vi "IRcam check.vi"() -> ()   [LabVIEW 2021]
uses:
  <vilib>/Platform/TimedLoop/XDataNode/timing_clust.ctl
  <vilib>/Platform/TimedLoop/XDataNode/nitl_modes.ctl
  <vilib>/Platform/TimedLoop/XDataNode/wakeup.ctl
  <vilib>/myRIO/Instrument Drivers/Onboard IO/I2C/typedefs/I2C User Configuration.ctl
  <vilib>/myRIO/Instrument Drivers/Onboard IO/I2C/typedefs/I2C Transfer Rate.ctl
  <vilib>/myRIO/Instrument Drivers/Onboard IO/I2C/typedefs/I2C Reference.ctl
  <vilib>/myRIO/Common/Instrument Driver Framework/Utilities/typedefs/myRIO Generic Hardware Reference.ctl
  <vilib>/myRIO/Common/Instrument Driver Framework/Utilities/typedefs/Hardware Version Enum.ctl
  <vilib>/myRIO/Common/Instrument Driver Framework/Utilities/typedefs/myRIO v1.0 Reference.ctl
  <vilib>/myRIO/Common/Instrument Driver Framework/Utilities/typedefs/Generic FPGA Reference.ctl
  <vilib>/myRIO/Common/Instrument Driver Framework/myRIO v1.0/I2C/typedefs/I2C Channels Enum.ctl
  <vilib>/myRIO/Instrument Drivers/Onboard IO/I2C/typedefs/I2C Configuration.ctl
  <vilib>/userDefined/High Color/nirio_resource_hc.ctl
  <vilib>/myRIO/Common/Instrument Driver Framework/Utilities/vis/Is FPGA Ref Available.vi
  <vilib>/myRIO/Common/Instrument Driver Framework/myRIO v1.0/I2C/vis/myRIO v1.1 Open I2C.vi
  <vilib>/myRIO/Instrument Drivers/Onboard IO/I2C/vis/Configure.vi
  <vilib>/myRIO/Instrument Drivers/Onboard IO/I2C/vis/Write.vi
  <vilib>/myRIO/Instrument Drivers/Onboard IO/I2C/vis/Write Read.vi
  <vilib>/myRIO/Common/Instrument Driver Framework/Utilities/vis/Validate Channels.vi
  <vilib>/myRIO/Common/Instrument Driver Framework/myRIO v1.0/I2C/vis/myRIO v1.0 Reserve I2C.vi
  <vilib>/myRIO/Common/Instrument Driver Framework/myRIO v1.0/I2C/vis/myRIO v1.0 Build MUX Configuration I2C.vi
  <vilib>/myRIO/Common/Instrument Driver Framework/myRIO v1.0/Resource Manager/vis/myRIO v1.0 Reserve Channel List.vi
  <vilib>/myRIO/Common/Instrument Driver Framework/myRIO v1.0/Resource Manager/vis/myRIO v1.0 Create Configuration List.vi
  <vilib>/myRIO/Common/Instrument Driver Framework/myRIO v1.0/Resource Manager/vis/myRIO v1.0 Reserve Channel.vi
  <vilib>/myRIO/Common/Instrument Driver Framework/myRIO v1.0/Resource Manager/vis/myRIO v1.0 Unreserve Channel.vi
  <vilib>/myRIO/Common/Instrument Driver Framework/myRIO v1.0/Resource Manager/vis/myRIO v1.0 Build Mutex Name.vi
  <vilib>/Utility/VariantDataType/GetNumericInfo.vi
  <vilib>/Utility/error.llb/Error Cluster From Error Code.vi
  <vilib>/myRIO/Common/Instrument Driver Framework/myRIO v1.0/myRIO v1.1 Open.vi
  <vilib>/myRIO/Common/Instrument Driver Framework/Utilities/vis/IO Manager.vi
  <vilib>/myRIO/Common/Instrument Driver Framework/Utilities/vis/Configuration Manager.vi
  <vilib>/myRIO/Common/Instrument Driver Framework/myRIO v1.0/Resource Manager/vis/myRIO v1.0 Configure IO.vi
  <vilib>/myRIO/Common/Instrument Driver Framework/myRIO v1.0/myRIO v1.0 Close.vi
  <vilib>/myRIO/Common/Instrument Driver Framework/myRIO v1.0/I2C/vis/myRIO v1.0 Configure I2C.vi
  <vilib>/myRIO/Common/Instrument Driver Framework/myRIO v1.0/I2C/vis/myRIO v1.0 Write I2C.vi
  <vilib>/myRIO/Common/Instrument Driver Framework/myRIO v1.0/I2C/vis/myRIO v1.0 Read I2C.vi
  <vilib>/platform/TimedLoop/XDataNode/XDataNode.xnode
  <vilib>/myRIO/Express VI/Onboard IO/I2C/I2C Express VI.xnode
  <vilib>/myRIO/Instrument Drivers/Onboard IO/I2C/vis/myRIO I2C Open.xnode
  <vilib>/Platform/TimedLoop/XDataNode/XDNodeRunTimeDep.lvlib
  <vilib>/myRIO/Instrument Drivers/Onboard IO/I2C/I2C.lvlib
panel:
  out "output":dbl format="%#_6f"
  out "output 2":dbl format="%#_6f"
  out "Decimal 2":i16 format="%0.0f"
  out "(hi.lo)":u16 format="%016b"
  out "Bytes Read":u8[](array[numeric]) format="%08b"
  in  "stop":bool
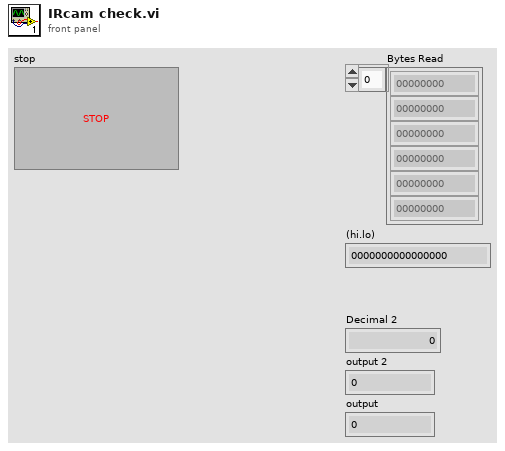
[diagram p1: front panel]
types:
  T1 = typedef "XDNodeRunTimeDep.lvlib/timing_clust.ctl" = cluster{"Expected End [f-1]":u64, "Actual End [f-1]":u64, "Finished Late? [f-1]":bool, "Expected End [i-1]":u64, "Actual End [i-1]":u64, "Finished Late? [i-1]":bool, "Expected Start [i]":u64, "Actual Start [i]":u64, "Expected Start [f]":u64, "Actual Start [f]":u64, "Source Name":string, "Structure Name":string, "Period":i64, "Deadline":i64, "Offset":i64, "Start":i64, "Priority":i32, "Timeout":i32, "Mode":T2, "Wakeup Reason":T3, "Error":errorcluster, "Source Type":string, "Secondary Source Type":string, "Global End Time":u64, "Global Start Time":u64, "Frame Duration":u64, "Iteration Duration":u64, "Assigned CPU":i32, "I/O Scan Engine Mode":u32}
  T2 = typedef "XDNodeRunTimeDep.lvlib/nitl_modes.ctl" = enum32{"No Change", "Process missed periods, maintain original phase", "Discard missed periods, maintain original phase", "Process missed periods, ignore original phase", "Discard missed periods, ignore original phase"}
  T3 = typedef "XDNodeRunTimeDep.lvlib/wakeup.ctl" = enum32{"Normal", "Aborted", "Asynchronous wakeup", "Timing source error", "Timed loop error", "Timeout"}
  T4 = typedef "I2C.lvlib/I2C Reference.ctl" = cluster{"myRIO Reference":T5, "I2C Channels Enum":T9, "I2C Configuration":T10}
  T5 = typedef "myRIO Generic Hardware Reference.ctl" = cluster{"myRIO Model":T6, "myRIO Hardware Reference":T7}
  T6 = typedef "Hardware Version Enum.ctl" = enum16{"Unknown", "myRIO-1900", "myRIO-1950", "roboRIO", "NI ELVIS RIO CM", "ELVIS III"}
  T7 = typedef "myRIO v1.0 Reference.ctl" = cluster{"Generic FPGA Reference":T8, "Allow multiple opens":bool}
  T8 = typedef "Generic FPGA Reference.ctl" = refnum<k20>
  T9 = typedef "I2C Channels Enum.ctl" = enum16{"Not Connected", "A/I2C", "B/I2C", "I2C/I2C"}
  T10 = typedef "I2C.lvlib/I2C Configuration.ctl" = cluster{"I2C Transfer Rate":T11}
  T11 = typedef "I2C.lvlib/I2C Transfer Rate.ctl" = enum16{"Standard mode (100 kbps)", "Fast mode (400 kbps)"}
  T12 = typedef "I2C.lvlib/I2C User Configuration.ctl" = cluster{"I2C Transfer Rate":T11}
  T13 = typedef "nirio_resource_hc.ctl" = tag
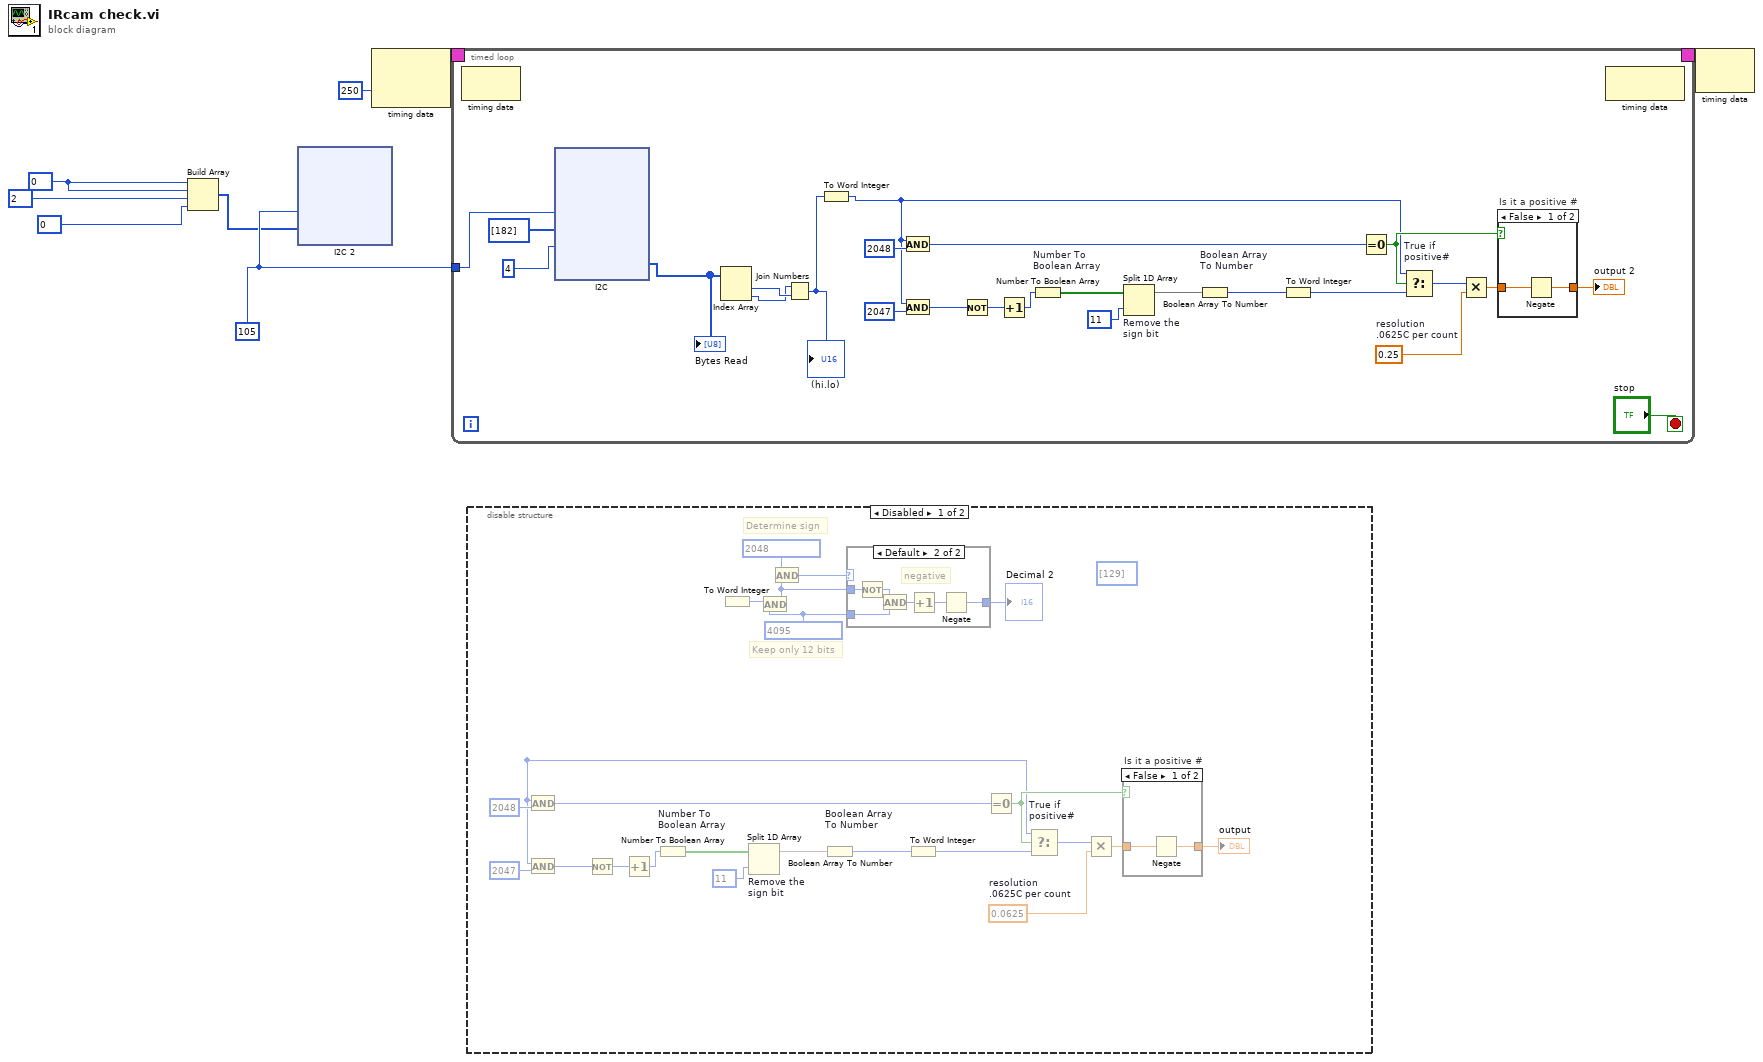
[diagram p0: block diagram]
diagram:
  w2 = u8 0
  w5 = u8 105 ("Slave Address (7-bit)")
  n1 = Build Array(w2, w2, u8 2, u8 0) -> (w4:u8[])
  n2 = xnode "I2C 2"("Slave Address (7-bit)"=w5, "Bytes to Write"=w4) -> ()  [unwired: 1 in, 1 out]
  n3 = node-c288(i64 250 ("Period")) -> (w8:T1)  [unwired: 1 in]
  n4 = timed-loop {
    timing: w8 -> [_]
    timing-out: [_] -> w7
    tunnel: w5 -> [w32]
    stop <- "stop" stop-if-true
    w28 = 0.25  # resolution .0625C per count
    n5 = node-c288() -> ()  [unwired: 1 in, 1 out]
    n6 = xnode "I2C"("Slave Address (7-bit)"=w32, "Bytes to Write"=u8[] [182], "Byte Count"=u32 4) -> ("Bytes Read"=w31:u8[])  [unwired: 1 in, 1 out]
    "Bytes Read" <- w31
    n7 = Index Array(array=w31) -> (element #1=w10:u8, element #2=w9:u8)  [unwired: 2 in]
    n8 = Join Numbers(hi=w9, lo=w10) -> ((hi.lo)=w11:u16)
    "(hi.lo)" <- w11
    n9 = To Word Integer(number=w11) -> (16bit integer=w12:i16)
    n10 = And ("Out = 0x800\nif neg #")(x=w12, y=u16 2048 ("number 2")) -> (x .and. y?=w25:u16)
    n11 = And ("Just the \n12 bits")(x=w12, y=i16 2047 ("number")) -> (x .and. y?=w14:i16)
    n12 = Not(x=w14) -> (.not. x?=w24:i16)
    n13 = Increment(x=w24) -> (x+1=w23:i16)
    n14 = Number To Boolean Array "Number To\nBoolean Array"(number=w23) -> (Boolean array=w22:bool[])
    n15 = Split 1D Array "Remove the \nsign bit"(array=w22, index=11) -> (first subarray=w15:bool[])  [unwired: 1 out]
    n16 = Boolean Array To Number "Boolean Array \nTo Number"(Boolean array=w15) -> (number=w20:u32)
    n17 = To Word Integer(number=w20) -> (16bit integer=w19:i16)
    n18 = Equal To 0?(x=w25) -> (x = 0?=w18:bool)
    n19 = Select "True if \npositive#"(t=w12, s=w18, f=w19) -> (s? t:f=w26:i16)
    n20 = Multiply(x=w26, y=w28) -> (x*y=w17:dbl)
    n21 = case "Is it a positive #" shown="False" w18 {
      tunnel: w17 -> [w35 w36]
      tunnel: [w34 w36] -> w16
      frame False {
        n22 = Negate(x=w35) -> (-x=w34:dbl)
      }
      frame True {
      }
    }
    "output 2" <- w16
    n23 = node-c288() -> ()  [unwired: 1 in, 1 out]
  }
  n24 = disable-structure shown="Disabled" {
    frame Disabled {
      w95 = 0.0625  # resolution .0625C per count
      w97 = i16 4095 ("Numeric")
      (unwired) u8[] [129] ("Bytes to Write")
      # "Determine sign"
      # "Keep only 12 bits"
      n25 = To Word Integer() -> (16bit integer=w96:i16)  [unwired: 1 in]
      n26 = And(x=w96, y=w97) -> (x .and. y?=w99:i16)
      n27 = And(x=i16 2048 ("Numeric"), y=w99) -> (x .and. y?=w100:i16)
      n28 = case shown="Default" w100 {
        tunnel: [w105 w106] -> w98
        tunnel: w99 -> [w105 w111]
        tunnel: w97 -> [_ w107]
        frame 0 {
          # "positive"
        }
        frame Default {
          # "negative"
          n29 = Not(x=w111) -> (.not. x?=w110:i16)
          n30 = And(x=w110, y=w107) -> (x .and. y?=w108:i16)
          n31 = Increment(x=w108) -> (x+1=w109:i16)
          n32 = Negate(x=w109) -> (-x=w106:i16)
        }
      }
      "Decimal 2" <- w98
      n33 = And ("Out = 0x800\nif neg #")(x=w79, y=u16 2048 ("number 2")) -> (x .and. y?=w92:u16)
      n34 = Equal To 0?(x=w92) -> (x = 0?=w85:bool)
      n35 = And ("Just the \n12 bits")(x=w79, y=i16 2047 ("number")) -> (x .and. y?=w81:i16)
      n36 = Not(x=w81) -> (.not. x?=w91:i16)
      n37 = Increment(x=w91) -> (x+1=w90:i16)
      n38 = Number To Boolean Array "Number To\nBoolean Array"(number=w90) -> (Boolean array=w89:bool[])
      n39 = Split 1D Array "Remove the \nsign bit"(array=w89, index=11) -> (first subarray=w82:bool[])  [unwired: 1 out]
      n40 = Boolean Array To Number "Boolean Array \nTo Number"(Boolean array=w82) -> (number=w87:u32)
      n41 = To Word Integer(number=w87) -> (16bit integer=w86:i16)
      n42 = Select "True if \npositive#"(s=w85, f=w86) -> (t=w79:i16, s? t:f=w93:i16)
      n43 = Multiply(x=w93, y=w95) -> (x*y=w84:dbl)
      n44 = case "Is it a positive #" shown="False" w85 {
        tunnel: w84 -> [w103 w104]
        tunnel: [w102 w104] -> w83
        frame False {
          n45 = Negate(x=w103) -> (-x=w102:dbl)
        }
        frame True {
        }
      }
      "output" <- w83
    }
    frame Enabled {
    }
  }
  n46 = node-c288(w7) -> ()  [unwired: 1 out]
